vi "Msg.vi"(7 "jettl in":refnum<class "jettl.lvclass">, 11 "Merge Error Msg Strategy in":refnum<class "Merge Error Msg Strategy.lvclass">) -> (5 "jettl out":refnum<class "jettl.lvclass">)   [LabVIEW 2021, in "jettl.lvlib" / "Merge Error.lvlib" / "Merge Error Msg Strategy.lvclass"]
uses:
  jettl/jettl/jettl.lvclass
  Merge Error Msg Strategy.lvclass
  Merge Error Msg Strategy.lvclass/Merge Error Msg Strategy.ctl
  Merge Error/Merge Error.lvclass
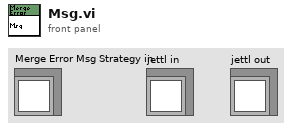
[diagram p1: front panel]
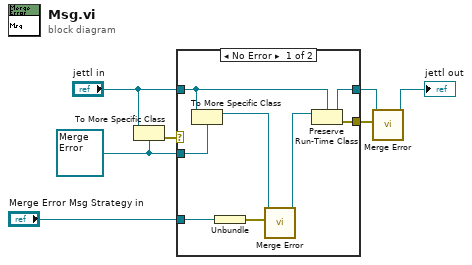
[diagram p0: block diagram]
diagram:
  w2 = refnum<class "Merge Error.lvclass"> refnum ("jettl.lvlib:Merge Error.lvlib:Merge Error.lvclass")
  n1 = To More Specific Class(target class=w2, reference="jettl in") -> (error out=w7:errorcluster)  [unwired: 1 in, 1 out]
  n2 = case shown="No Error" w7 {
    selector: w7 -> [_ w16]
    tunnel: [w13 w17] -> w5
    tunnel: "jettl in" -> [w14 w17]
    tunnel: w2 -> [w15 _]
    tunnel: [w12 w16] -> w6
    tunnel: "Merge Error Msg Strategy in" -> [w9 _]
    frame No Error {
      n3 = To More Specific Class(target class=w15, reference=w14) -> (specific class reference=w11:refnum<class "Merge Error.lvclass">)  [unwired: 1 in, 1 out]
      n4 = Unbundle(w9) -> (w8:errorcluster)
      n5 = call-dynamic "Merge Error.vi"("Error"=w8, "Merge Error in"=w11) -> ("Merge Error out"=w10:refnum<class "Merge Error.lvclass">)  [unwired: 9 in]
      n6 = Preserve Run-Time Class(object in=w10, 2:w14) -> (object out=w13:refnum<class "jettl.lvclass">, error out=w12:errorcluster)  [unwired: 1 in]
    }
    frame Error {
    }
  }
  n7 = call-dynamic "Merge Error.vi"("Error"=w6, "jettl in"=w5) -> ("jettl out"=→"jettl out":refnum<class "jettl.lvclass">)  [unwired: 9 in]
